vi "FV-split_data_up.vi"(11 "split data":T2) -> (3 "split data 2":T2)   [LabVIEW 2020, in "FV-file_viewer.lvlib"]
uses:
  FV-file_viewer.lvlib
  FV-splitting_data.ctl
  record_file_handler/VFH-file_cluster-R140.ctl
  record_file_handler/VFH-file_cluster-NanoVNA.ctl
  FV-water_cluster.ctl
  FV-single_XY_plot.ctl
  record_file_handler/VFH-VNA_File_Handler.lvlib
panel:
  out "First Part":T1
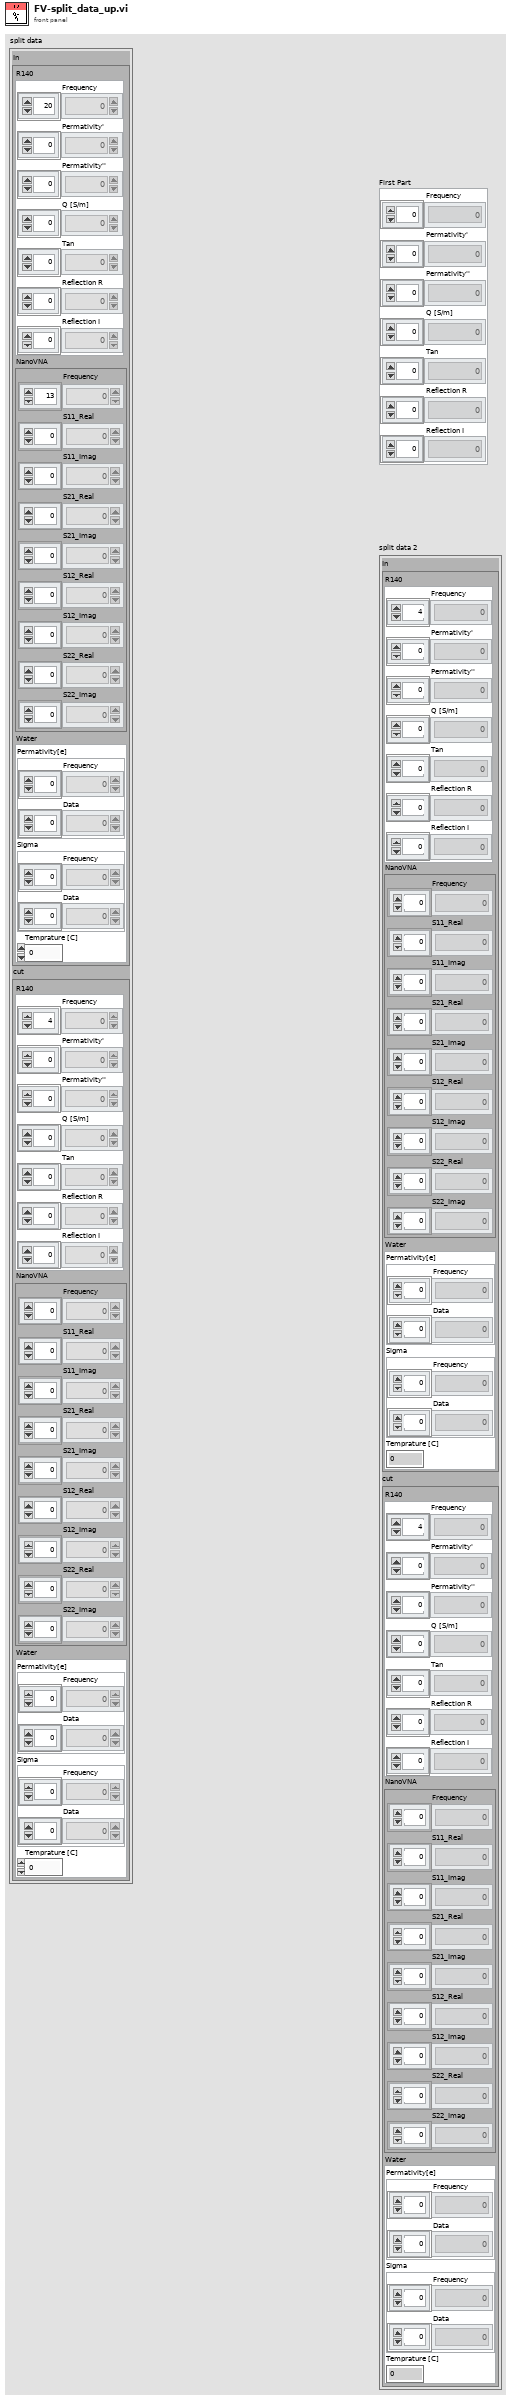
[diagram p1: front panel]
types:
  T1 = typedef "VFH-VNA_File_Handler.lvlib/VFH-file_cluster-R140.ctl" = cluster{"Frequency":dbl[], "Permativity'":dbl[], "Permativity''":dbl[], "Q [S/m]":dbl[], "Tan":dbl[], "Reflection R":dbl[], "Reflection I":dbl[]}
  T2 = typedef "FV-file_viewer.lvlib/FV-splitting_data.ctl" = cluster{"In":cluster{"R140":T1, "NanoVNA":T3, "Water":T4}, "cut":cluster{"R140":T1, "NanoVNA":T3, "Water":T4}}
  T3 = typedef "VFH-VNA_File_Handler.lvlib/VFH-file_cluster-NanoVNA.ctl" = cluster{"Frequency":dbl[], "S11_Real":dbl[], "S11_Imag":dbl[], "S21_Real":dbl[], "S21_Imag":dbl[], "S12_Real":dbl[], "S12_Imag":dbl[], "S22_Real":dbl[], "S22_Imag":dbl[]}
  T4 = typedef "FV-file_viewer.lvlib/FV-water_cluster.ctl" = cluster{"Permativity[e]":T5, "Sigma":T5, "Temprature [C]":dbl}
  T5 = typedef "FV-file_viewer.lvlib/FV-single_XY_plot.ctl" = cluster{"Frequency":dbl[], "Data":dbl[]}
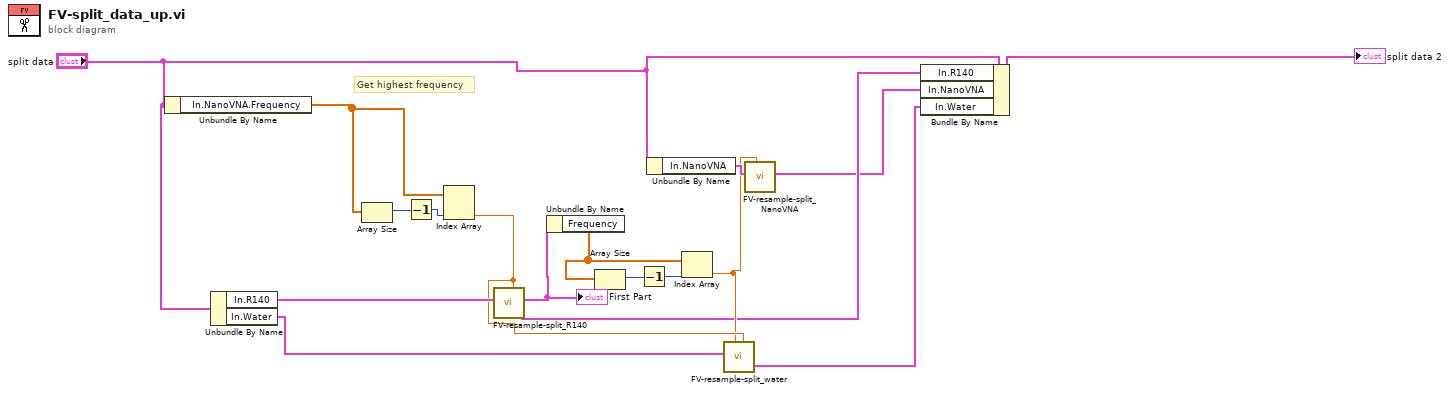
[diagram p0: block diagram]
diagram:
  # "Get highest frequency"
  n1 = Unbundle By Name("split data") -> ("In.NanoVNA.Frequency"=w16:dbl[])
  n2 = Unbundle By Name("split data") -> ("In.R140"=w15:T1, "In.Water"=w14:T4)
  n3 = Array Size(array=w16) -> (size(s)=w17:i32)
  n4 = Decrement(x=w17) -> (x-1=w13:i32)
  n5 = Index Array(array=w16, index #2=w13) -> (element #2=w12:dbl)  [unwired: 1 in, 1 out]
  n6 = call "FV-resample-split_R140.vi"("Max Frequency"=w12, "R140"=w15) -> ("Second Part"=w3:T1, "First Part"=w10:T1)  [unwired: 8 in]
  "First Part" <- w10
  n7 = Unbundle By Name(w10) -> ("Frequency"=w8:dbl[])
  n8 = Array Size(array=w8) -> (size(s)=w9:i32)
  n9 = Decrement(x=w9) -> (x-1=w6:i32)
  n10 = Unbundle By Name("split data") -> ("In.NanoVNA"=w7:T3)
  n11 = Index Array(array=w8, index=w6) -> (element=w5:dbl)
  n12 = call "FV-resample-split_water.vi"("Max Frequency"=w12, "min Frequency"=w5, "water"=w14) -> ("water out"=w1:T4)  [unwired: 8 in]
  n13 = call "FV-resample-split_NanoVNA.vi"("min Frequency"=w5, "NanoVNA"=w7) -> ("output cluster"=w2:T3)  [unwired: 9 in]
  n14 = Bundle By Name(cluster="split data", "In.R140"=w3, "In.NanoVNA"=w2, "In.Water"=w1) -> (→"split data 2":T2)
